vi "Capacitance Estimator.vi"(1 "normalized waveform":waveform(dbl)={"t0"=timestamp(3087922235.213 s since 1904-01-01), "dt"=1.9999999494757503e-05, "Y"=array[1000 elements]}, 2 "Resistance (Ohms)":dbl=100000.0 format="%.4e") -> (0 "Estimated Capacitance (F)":dbl=1.269612045289484e-08 format="%.4e")   [LabVIEW 2016]
doc: "Given an RC decay waveform and the resistance R, this vi estimates the capacitance by determining the 1/e time.\n\nPaul K Dixon\nPhysics 350\nCSUSB Physics"
panel:
  # "C(T) Capacitance Estimator"
  # "1.2696E-8"
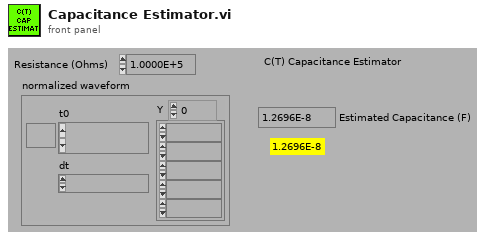
[diagram p1: front panel]
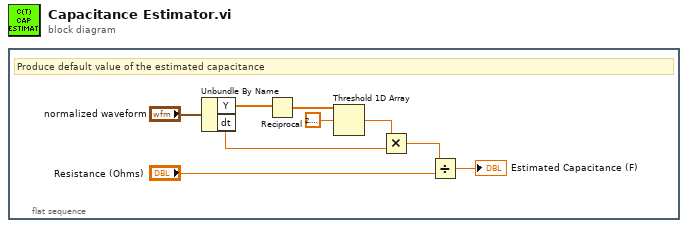
[diagram p0: block diagram]
diagram:
  n1 = flat-sequence {
    frame #0 {
      # "Produce default value of the estimated capacitance"
      n2 = Unbundle By Name("normalized waveform") -> ("Y"=w8:dbl[], "dt"=w4:dbl)
      n3 = Reciprocal(x=w8) -> (1/x=w7:dbl[])
      n4 = Threshold 1D Array(2:2.718281828459045, 3:w7) -> (0:w5:dbl)  [unwired: 1 out]
      n5 = Multiply(x=w5, y=w4) -> (x*y=w3:dbl)
      n6 = Divide(x=w3, y="Resistance (Ohms)") -> (x/y=→"Estimated Capacitance (F)":dbl)
    }
  }
